vi "Create Channels.vi"(8 "error in (no error)":errorcluster, 10 "Channels to Create in":T1[](array[typedef]) {"Type" items=["CIFTag_Double"=100, "CIFTag_U64"=101, "CIFTag_I64"=102]}, 11 "CIFCorePlugin in":refnum<class "CIFCorePlugin.lvclass">) -> (0 "error out":errorcluster, 2 "Channels to Create out":T1[](array[typedef]) {"Type" items=["CIFTag_Double"=100, "CIFTag_U64"=101, "CIFTag_I64"=102]}, 3 "CIFCorePlugin out":refnum<class "CIFCorePlugin.lvclass">)   [LabVIEW 2021, in "CIFCorePlugin.lvclass"]
uses:
  CIFCorePlugin.lvclass
  CIFCorePlugin.lvclass/CIFCorePlugin.ctl
  Channels/ChannelRegistrar/ChannelRegistrar.lvlib
  CIFUtilities/CIFChannels/Typedef/Direction.ctl
  CIFUtilities/CIFChannels/CIFChannels.lvclass
  Channels/ChannelRegistrar/typedef/Registered Channel Types.ctl
  Channels/ChannelRegistrar/typedef/Channel Definition.ctl
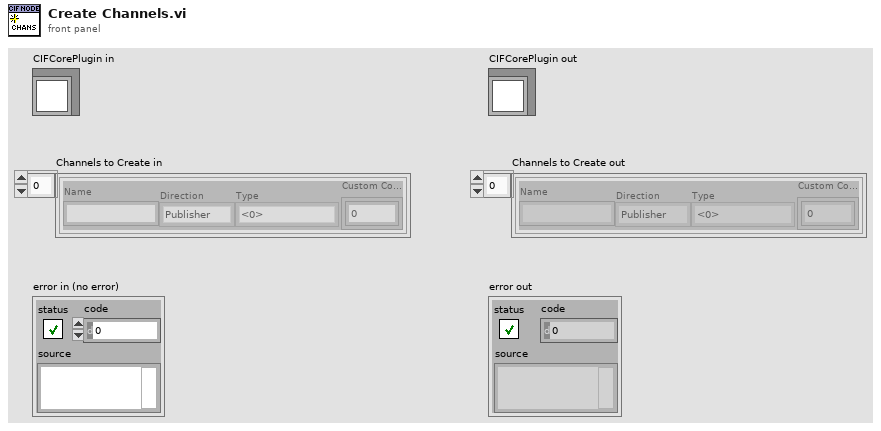
[diagram p1: front panel]
types:
  T1 = typedef "ChannelRegistrar.lvlib/Channel Definition.ctl" = cluster{"Name":string, "Direction":T2, "Type":T3, "Custom Config Data":u8[]}
  T2 = typedef "CIFChannels.lvclass/Direction.ctl" = enum16{"Publisher", "Subscriber"}
  T3 = typedef "ChannelRegistrar.lvlib/Registered Channel Types.ctl" = u16
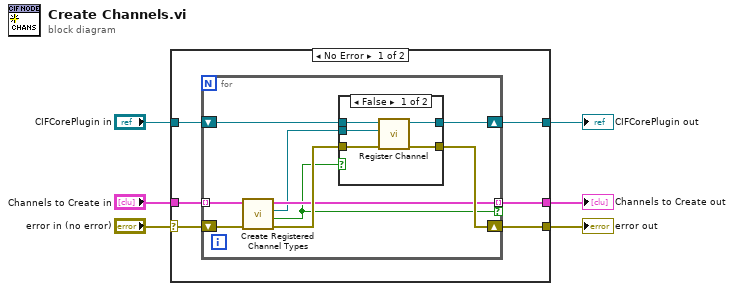
[diagram p0: block diagram]
diagram:
  n1 = case shown="No Error" "error in (no error)" {
    selector: "error in (no error)" -> [w11 w31]
    tunnel: [w9 w31] -> w5
    tunnel: [w10 w30] -> w3
    tunnel: "CIFCorePlugin in" -> [w12 w30]
    tunnel: "Channels to Create in" -> [w8 w29]
    tunnel: [w7 w29] -> w1
    frame No Error {
      n2 = for {
        tunnel: w8 -> [w17] mode=indexing
        shift-right: [w20] -> w10
        shift-left: w12 -> [w21]
        shift-right: [w18] -> w9
        shift-left: w11 -> [w19]
        tunnel: [w15] -> w7 mode=indexing if=w13
        n3 = call "Create Registered Channel Types.vi"("error in"=w19, "Channel Definition in"=w17) -> ("error out"=w16:errorcluster, "Not Registered"=w13:bool, "Channel out"=w14:refnum<class "CIFChannels.lvclass">, "Channel Definition out"=w15:T1)  [unwired: 6 in]
        n4 = case shown="False" w13 {
          tunnel: w21 -> [w26 w28]
          tunnel: [w25 w28] -> w20
          tunnel: [w24 w27] -> w18
          tunnel: w16 -> [w23 w27]
          tunnel: w14 -> [w22 _]
          frame False {
            n5 = call "Register Channel.vi"("error in (no error)"=w23, "Channel"=w22, "CIFCorePlugin in"=w26) -> ("error out"=w24:errorcluster, "CIFCorePlugin out"=w25:refnum<class "CIFCorePlugin.lvclass">)  [unwired: 7 in]
          }
          frame True {
          }
        }
      }
    }
    frame Error {
    }
  }
  "error out" <- w5
  "CIFCorePlugin out" <- w3
  "Channels to Create out" <- w1
